vi "TMCM351-ReadAnalogIOAll.vi"(4 "错误输入":errorcluster caption="错误输入（无错误）", 7 "com in":refnum<visa-resource-name>) -> (0 "错误输出":errorcluster, 2 "AnalogOut":i32[](array[numeric]), 3 "comOut":refnum<visa-resource-name>)   [LabVIEW 2018]
panel:
  # "读取IO口"
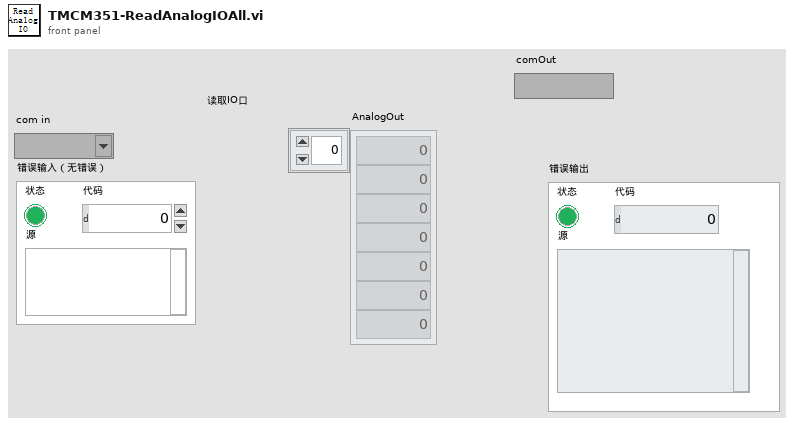
[diagram p1: front panel]
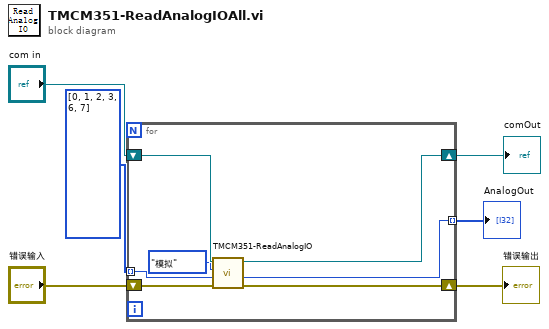
[diagram p0: block diagram]
diagram:
  n1 = for {
    tunnel: i32[] [0, 1, 2, 3, 6, 7] -> [w8] mode=indexing
    tunnel: [w12] -> w1 mode=indexing
    shift-right: [w11] -> w2
    shift-left: "com in" -> [w13]
    shift-right: [w7] -> w3
    shift-left: "错误输入" -> [w10]
    n2 = call "TMCM351-ReadAnalogIO.vi"("错误输入"=w10, "通道"=w8, "数据源"=enum8{"数字", "模拟"}."模拟", "com in"=w13) -> ("错误输出"=w7:errorcluster, "ReadOut"=w12:i32, "com out"=w11:refnum<visa-resource-name>)  [unwired: 1 in]
  }
  "错误输出" <- w3
  "comOut" <- w2
  "AnalogOut" <- w1
